vi "ni579x Config FPGA Template.vi"() -> ()   [LabVIEW 2012]
uses:
  <vilib>/Platform/TimedLoop/XDataNode/wakeup.ctl
  <vilib>/Platform/TimedLoop/XDataNode/XDNodeRunTimeDep.lvlib
  <vilib>/Platform/TimedLoop/XDataNode/nitl_modes.ctl
  <vilib>/Platform/TimedLoop/XDataNode/timing_clust.ctl
  <vilib>/Platform/TimedLoop/XDataNode/XDataNode.xnode
  <instrlib>/ni579x/Register Bus/v1/FPGA/ni579x Register Bus v1 FPGA.lvlib
  <vilib>/eio/EIONode/EIONode.xnode
  <instrlib>/ni579x/Register Bus/v1/FPGA/Private/Mux/Read Completion Mux (3 inputs).vi
  <instrlib>/ni579x/Synchronization/v1/FPGA/ni579x Synchronization v1 FPGA.lvlib
  <vilib>/rvi/eio/common/nirviEmuTemplateMethod_errors.vi
  <instrlib>/ni579x/Register Bus/v1/FPGA/Public/Read Cmd Data.ctl
panel:
  in  "reg.host read.go rcvd 0":bool
  out "reg.notify host.go 0":bool
  in  "reg.notify host.go rcvd 0":bool
  out "reg.host read.data 0":T1
  in  "reg.reset 0":bool
  out "IO Module\\Initialization Done":bool
  out "IO Module\\PLL Locked":bool
  out "IO Module\\LO Locked":bool
  out "IO Module\\User Error":u8
  # "REGISTER BUS"
  # "Required Controls & Indicators"
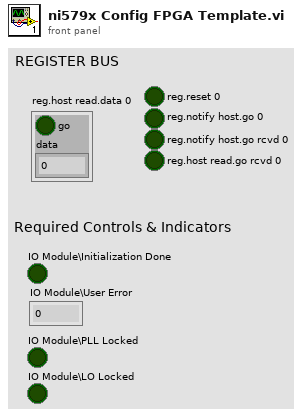
[diagram p1: front panel]
types:
  T1 = typedef "ni579x Register Bus v1 FPGA.lvlib/Read Cmd Data.ctl" = cluster{"go":bool, "data":u32}
  T2 = typedef "XDNodeRunTimeDep.lvlib/timing_clust.ctl" = cluster{"Expected End [f-1]":u64, "Actual End [f-1]":u64, "Finished Late? [f-1]":bool, "Expected End [i-1]":u64, "Actual End [i-1]":u64, "Finished Late? [i-1]":bool, "Expected Start [i]":u64, "Actual Start [i]":u64, "Expected Start [f]":u64, "Actual Start [f]":u64, "Source Name":string, "Structure Name":string, "Period":i64, "Deadline":i64, "Offset":i64, "Start":i64, "Priority":i32, "Timeout":i32, "Mode":T3, "Wakeup Reason":T4, "Error":errorcluster, "Source Type":string, "Secondary Source Type":string, "Global End Time":u64, "Global Start Time":u64, "Frame Duration":u64, "Iteration Duration":u64, "Assigned CPU":i32, "I/O Scan Engine Mode":u32}
  T3 = typedef "XDNodeRunTimeDep.lvlib/nitl_modes.ctl" = enum32{"No Change", "Process missed periods, maintain original phase", "Discard missed periods, maintain original phase", "Process missed periods, ignore original phase", "Discard missed periods, ignore original phase"}
  T4 = typedef "XDNodeRunTimeDep.lvlib/wakeup.ctl" = enum32{"Normal", "Aborted", "Asynchronous wakeup", "Timing source error", "Timed loop error", "Timeout"}
  T5 = typedef "ni579x Synchronization v1 FPGA.lvlib/resources.ctl" = cluster{"master":refnum<k21>, "meas.enable":refnum<k21>, "meas.ready":refnum<k21>, "meas.arm":refnum<k21>, "meas.valid":refnum<k21>, "meas.value":refnum<k21>, "cptr":refnum<k21>, "cptr.adjust":refnum<k21>, "cptr.period":refnum<k21>}
  T6 = typedef "ni579x Register Bus v1 FPGA.lvlib/Register Instruction.ctl" = cluster{"subsystem":u8, "address":u16, "data":u32, "valid":bool, "read":bool}
  T7 = typedef "ni579x Register Bus v1 FPGA.lvlib/Read Completion.ctl" = cluster{"data":u32, "valid":bool}
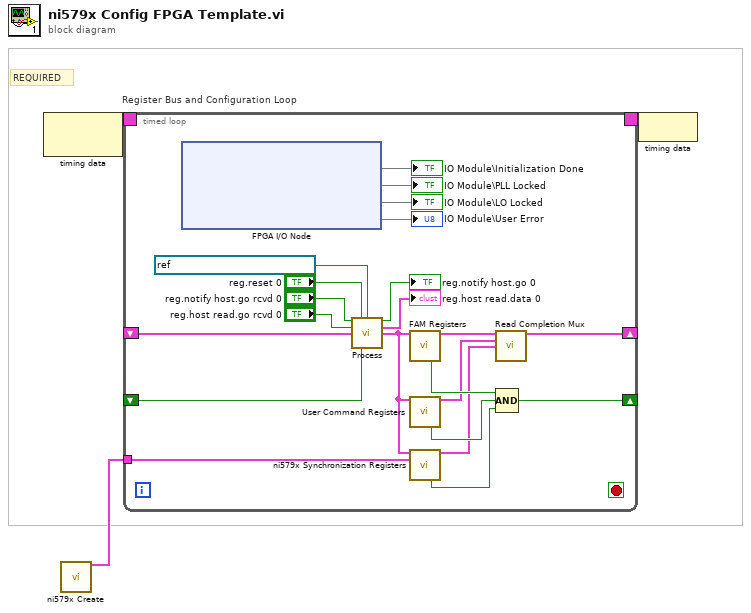
[diagram p0: block diagram]
diagram:
  # "REQUIRED"
  n1 = node-c288() -> (w3:T2)  [unwired: 1 in]
  n2 = call <instrlib>:"ni579x Create.vi"() -> ("sync.resources"=w1:T5)  [unwired: 15 in]
  n3 = timed-loop "Register Bus and Configuration Loop" {
    timing: w3 -> [_]
    timing-out: [_] -> w2
    shift-right: [w18] -> _
    shift-left: _ -> [w17]
    shift-right: [w16] -> _
    shift-left: _ -> [w15]
    tunnel: w1 -> [w4]
    stop <- _ stop-if-true
    n4 = xnode "FPGA I/O Node"() -> ("IO Module\\Initialization Done"=→"IO Module\\Initialization Done", "IO Module\\PLL Locked"=→"IO Module\\PLL Locked", "IO Module\\LO Locked"=→"IO Module\\LO Locked", "IO Module\\User Error"=→"IO Module\\User Error")  [unwired: 4 in, 4 out]
    n5 = call <instrlib>:"Process.vi"("reg.notify host.go rcvd"="reg.notify host.go rcvd 0", "reg.reset"="reg.reset 0", "reg.host instruction fifo"=refnum<k21> "reg.host instruction fifo 0", "reg.host read.go rcvd"="reg.host read.go rcvd 0", "read completion"=w17, "ready for output"=w15) -> ("reg.notify host.go"=→"reg.notify host.go 0":bool, "reg.host read.data"=→"reg.host read.data 0":T1, "register instruction"=w7:T6)  [unwired: 7 in]
    n6 = call <instrlib>:"FAM Registers.vi"("register instruction"=w7) -> ("read completion"=w20:T7, "ready for input"=w22:bool)  [unwired: 12 in, 1 out]
    n7 = call <instrlib>:"User Command Registers.vi"("register instruction"=w7) -> ("read completion"=w19:T7, "ready for input"=w21:bool)  [unwired: 11 in, 2 out]
    n8 = call <instrlib>:"ni579x Synchronization Registers.vi"("register instruction"=w7, "sync.resources"=w4) -> ("read completion"=w6:T7, "ready for input"=w5:bool)  [unwired: 12 in]
    n9 = call-poly <instrlib>:"Read Completion Mux.vi"("element 0"=w20, "element 1"=w19, "element 2"=w6) -> ("read completion out"=w18:T7)  [unwired: 12 in]
    n10 = Compound Arithmetic op=AND(w22, w21, w5) -> (w16:bool)
  }
  n11 = node-c288(w2) -> ()
